vi "Initialize.vi"(7 "Timeout (3 sec)":dbl=3.0 format="%.2f", 8 "error in (no error)":errorcluster, 9 "Reset (T)":bool=TRUE, 10 "ID Query (T)":bool=TRUE, 11 "VISA name":refnum<visa-resource-name>) -> (0 "error out":errorcluster, 3 "VISA out":refnum<visa-resource-name>)   [LabVIEW 2025, in "TDK-Lambda GEN LAN Series.lvlib"]
doc: "Establishes communication with the instrument. You must run this VI before using any other driver VIs for this instrument. Generally, you need to call the Initialize VI only once at the beginning of an application.\n\nYou may optionally reset the instrument and/or verify ithe instrument identity starts with \"LAMBDA,GEN...\"."
uses:
  <userlib>/TDK-Lambda GEN LAN Series/TDK-Lambda GEN LAN Series.lvlib
panel:
  # "Initialize Instrument\nOpen VISA Port"
  # "TDK-Lambda Genesys \n  LAN\n  DC Power Supplies"
  # "Seconds"
  # "(c) 2019 TDK-Lambda.  ALL RIGHTS RESERVED."
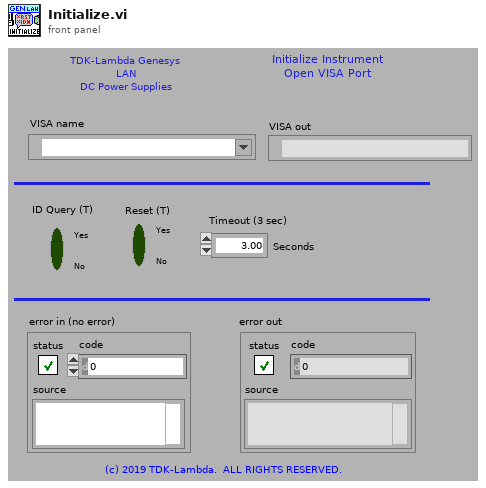
[diagram p1: front panel]
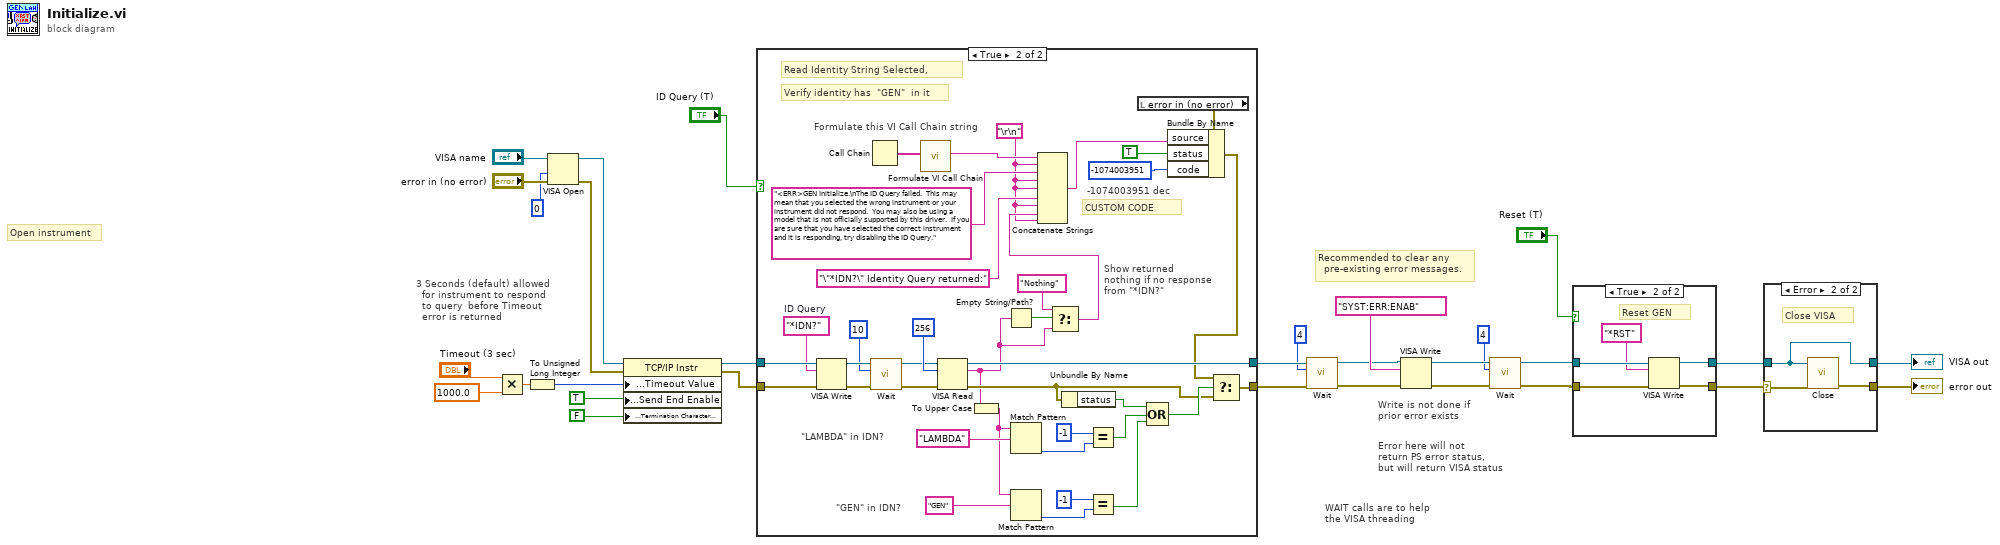
[diagram p0: block diagram]
diagram:
  # "WAIT calls are to help\nthe VISA threading"
  # "Error here will not\nreturn PS error status,\nbut will return VISA status"
  # "Write is not done if\nprior error exists"
  # "Recommended to clear any  \n  pre-existing error messages."
  # "3 Seconds (default) allowed\n  for instrument to respond \n  to query  before Timeout\n  error is returned"
  # "Open instrument"
  n1 = Multiply(x="Timeout (3 sec)", y=1000.0) -> (x*y=w17:dbl)
  n2 = To Unsigned Long Integer(number=w17) -> (unsigned 32bit integer=w6:u32)
  n3 = VISA Open(access mode=u32 0, error in (no error)="error in (no error)", VISA resource name="VISA name") -> (VISA resource name=w8:refnum<visa-resource-name>, error out=w7:errorcluster)  [unwired: 2 in]
  n4 = property class="TCP/IP Instr"(reference=w8, error in=w7, "General Settings:Timeout Value"=w6, "Message Based Settings:Send End Enable"=TRUE, "Message Based Settings:Termination Character Enable"=FALSE ("Message Based Settings:Send End Enable")) -> (reference out=w22:refnum<visa-resource-name>, error out=w21:errorcluster)
  n5 = case shown="True" "ID Query (T)" {
    tunnel: [w31 w69] -> w11
    tunnel: [w32 w66] -> w13
    tunnel: w22 -> [w32 w67]
    tunnel: w21 -> [w31 w68]
    frame False {
      # "Do Not Read Identity String"
    }
    frame True {
      w33 = "\r\n"
      w61 = "*IDN?"  # ID Query
      # "Show returned\nnothing if no response\nfrom \"*IDN?\""
      # "Formulate this VI Call Chain string"
      # "-1074003951 dec"
      # "CUSTOM CODE"
      # "\"GEN\" in IDN?"
      # "\"LAMBDA\" in IDN?"
      # "Verify identity has  \"GEN\"  in it"
      # "Read Identity String Selected,"
      n6 = VISA Write(VISA resource name=w67, write buffer=w61, error in (no error)=w68) -> (VISA resource name out=w40:refnum<visa-resource-name>, error out=w38:errorcluster)  [unwired: 1 out]
      n7 = Call Chain() -> (call chain=w34:string[])
      n8 = call <userlib>:"Wait.vi"("error"=w38, "Delay (20 mS)"=u32 10, "VISA"=w40) -> ("error out"=w37:errorcluster, "VISA out"=w39:refnum<visa-resource-name>)  [unwired: 7 in]
      n9 = call <userlib>:"Formulate VI Call Chain.vi"("Call Chain"=w34) -> ("String Out"=w35:string)  [unwired: 10 in]
      n10 = VISA Read(VISA resource name=w39, byte count=u32 256, error in (no error)=w37) -> (VISA resource name out=w66:refnum<visa-resource-name>, read buffer=w42:string, error out=w53:errorcluster)  [unwired: 1 out]
      n11 = To Upper Case(1:w42) -> (0:w41:string)
      n12 = Empty String/Path?(string/path=w42) -> (empty?=w45:bool)
      n13 = Match Pattern(string=w41, regular expression="LAMBDA") -> (offset past match=w63:i32)  [unwired: 1 in, 3 out]
      n14 = Match Pattern(string=w41, regular expression="GEN") -> (offset past match=w60:i32)  [unwired: 1 in, 3 out]
      n15 = Select(t="Nothing" ("Source"), s=w45, f=w42) -> (s? t:f=w43:string)
      n16 = Concatenate Strings(w35, w33, "<ERR>GEN Initialize.\nThe ID Query failed.  This may mean that you selected the wrong instrument or your instrument did not respond.  You may also be using a model that is not officially supported by this driver.  If you are sure that you have selected the correct instrument and it is responding, try disabling the ID Query." ("Source (VI Name)"), w33, w33, "\"*IDN?\" Identity Query returned:" ("Source"), w33, w43, w33) -> (w48:string)
      n17 = Unbundle By Name(w53) -> ("status"=w57:bool)
      n18 = Equal?(x=-1, y=w63) -> (x = y?=w56:bool)
      n19 = Equal?(x=-1, y=w60) -> (x = y?=w55:bool)
      n20 = local read "error in (no error)"() -> (w49:errorcluster)
      n21 = Compound Arithmetic op=OR(w57, w56, w55) -> (w54:bool)
      n22 = Bundle By Name(cluster=w49, "source"=w48, "status"=TRUE, "code"=-1074003951) -> (w47:errorcluster)
      n23 = Select(t=w47, s=w54, f=w53) -> (s? t:f=w69:errorcluster)
    }
  }
  n24 = call <userlib>:"Wait.vi"("error"=w11, "Delay (20 mS)"=u32 4, "VISA"=w13) -> ("error out"=w10:errorcluster, "VISA out"=w12:refnum<visa-resource-name>)  [unwired: 7 in]
  n25 = VISA Write(VISA resource name=w12, write buffer="SYST:ERR:ENAB", error in (no error)=w10) -> (VISA resource name out=w5:refnum<visa-resource-name>, error out=w4:errorcluster)  [unwired: 1 out]
  n26 = call <userlib>:"Wait.vi"("error"=w4, "Delay (20 mS)"=u32 4, "VISA"=w5) -> ("error out"=w3:errorcluster, "VISA out"=w2:refnum<visa-resource-name>)  [unwired: 7 in]
  n27 = case shown="True" "Reset (T)" {
    tunnel: w3 -> [w70 w74]
    tunnel: [w70 w72] -> w20
    tunnel: w2 -> [w71 w76]
    tunnel: [w71 w75] -> w28
    frame False {
      # "Do Not\n  Reset"
    }
    frame True {
      # "Reset GEN"
      n28 = VISA Write(VISA resource name=w76, write buffer="*RST", error in (no error)=w74) -> (VISA resource name out=w75:refnum<visa-resource-name>, error out=w72:errorcluster)  [unwired: 1 out]
    }
  }
  n29 = case shown="Error" w20 {
    selector: w20 -> [w77 w81]
    tunnel: w28 -> [w78 w79]
    tunnel: [w78 w79] -> w27
    tunnel: [w77 w80] -> w26
    frame No Error {
    }
    frame Error {
      # "Close VISA"
      n30 = call "Close.vi"("error"=w81, "VISA name"=w79) -> ("error out"=w80:errorcluster)  [unwired: 9 in]
    }
  }
  "VISA out" <- w27
  "error out" <- w26
